vi "Get Type Code.vi"(8 "error in (no error)":errorcluster, 11 "LVType.lvclass in":refnum<class "LVType.lvclass">) -> (0 "error out":errorcluster, 1 "TypeCodeString":string, 2 "Type":T1, 3 "LVType.lvclass out":refnum<class "LVType.lvclass">)   [LabVIEW 2020, in "LVDataTypes.lvlib" / "LVType.lvclass"]
uses:
  <vilib>/AppBuilder/Engine/WebServiceDescription/LVDataTypes/LVType/LVType.lvclass
  <vilib>/AppBuilder/Engine/WebServiceDescription/LVDataTypes/TypeCode.ctl
  <vilib>/AppBuilder/Engine/WebServiceDescription/LVDataTypes/LVType/LVType.lvclass/LVType.ctl
  <vilib>/AppBuilder/Engine/WebServiceDescription/LVDataTypes/LVDataTypes.lvlib
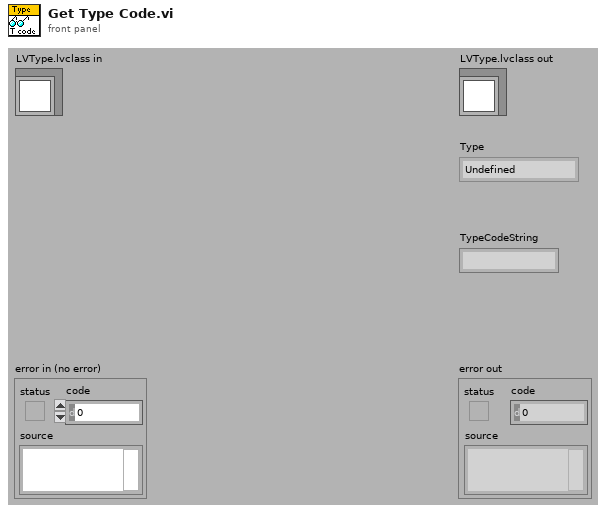
[diagram p1: front panel]
types:
  T1 = typedef "LVDataTypes.lvlib/TypeCode.ctl" = enum16{"Undefined", "Byte", "Unsigned Byte", "Word", "Unsigned Word", "Long", "Unsigned Long", "Quad", "Unsigned Quad", "Single", "Double", "Extended", "Enum", "Boolean", "String", "Path", "Array", "Cluster", "AnalogWaveform", "DigitalWaveform", "Time Stamp", "Void", "Complex Single", "Complex Double", "Complex Extended"}
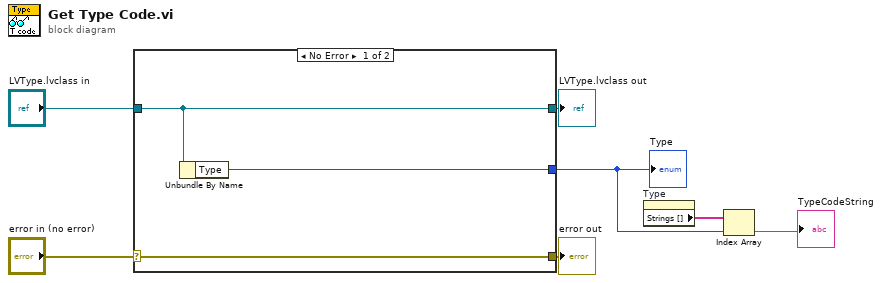
[diagram p0: block diagram]
diagram:
  n1 = case shown="No Error" "error in (no error)" {
    selector: "error in (no error)" -> [w10 w11]
    tunnel: [w10 w11] -> w6
    tunnel: [w9 w12] -> w4
    tunnel: "LVType.lvclass in" -> [w9 w12]
    tunnel: [w8 _] -> w2
    frame No Error {
      n2 = Unbundle By Name(w9) -> ("Type"=w8:T1)
    }
    frame Error {
    }
  }
  "error out" <- w6
  "LVType.lvclass out" <- w4
  "Type" <- w2
  n3 = property on="Type" class="Enum (strict)"() -> ("Strings []"=w3:string[])  [unwired: 2 in, 2 out]
  n4 = Index Array(array=w3, index=w2) -> (element=→"TypeCodeString":string)
